vi "OnResize2.vi"(0 "XRef":T15, 1 "Bounds":T13, 2 "Mouse Mods":T11, 3 "State In":T1) -> (14 "Reply":T9, 15 "Fatal Error Out":T8, 16 "State Out":T1)   [LabVIEW 2020, in "Parallel Diagram Block.xnode"]
uses:
  Parallel Diagram Block.xnode
  <vilib>/XNodeSupport/XNodeInt.ctl
  <vilib>/XNodeSupport/NI_XNodeSupport.lvlib
  <vilib>/XNodeSupport/XNodeString.ctl
  <vilib>/XNodeSupport/XNodeStringArray.ctl
  <vilib>/XNodeSupport/XNodeXNodeRef.ctl
  <vilib>/XNodeSupport/XNodeRect32.ctl
  <vilib>/XNodeSupport/XNodeBool.ctl
  <vilib>/XNodeSupport/XNodeMouseMods.ctl
  <vilib>/XNodeSupport/XNodeErrorCluster.ctl
  State.ctl
  Parallel Block/Value Type.ctl
  Parallel Block/Parallel Block.lvlib
  Parallel Block/Type Descriptor.ctl
  <vilib>/picture/picture.llb/imagedata.ctl
  Parallel Block/Direction.ctl
  Parallel Block/Terminal Mode.ctl
  Parallel Block/Terminal Type.ctl
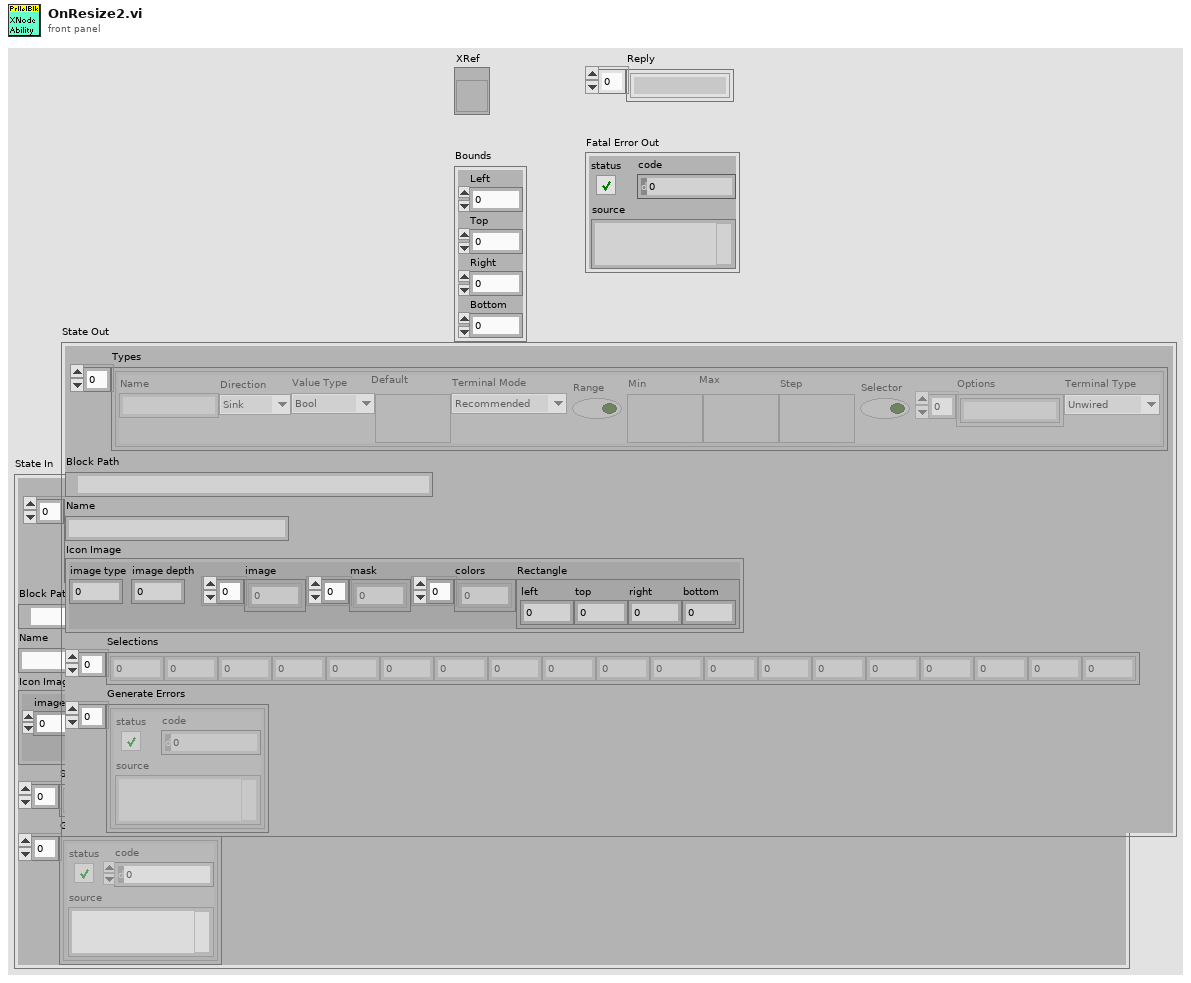
[diagram p1: front panel]
types:
  T1 = typedef "Parallel Diagram Block.xnode/State.ctl" = cluster{"Types":T2[], "Block Path":path, "Name":string, "Icon Image":T7, "Selections":i32[], "Generate Errors":errorcluster[]}
  T2 = typedef "Parallel Block.lvlib/Type Descriptor.ctl" = cluster{"Name":string, "Direction":T3, "Value Type":T4, "Default":variant, "Terminal Mode":T5, "Range":bool, "Min":variant, "Max":variant, "Step":variant, "Selector":bool, "Options":string[], "Terminal Type":T6}
  T3 = typedef "Parallel Block.lvlib/Direction.ctl" = enum16{"Sink", "Source"}
  T4 = typedef "Parallel Block.lvlib/Value Type.ctl" = enum16{"Unknown", "Bool", "U8", "U16", "U32", "U64", "I8", "I16", "I32", "I64", "SGL", "DBL", "CSG", "CDB", "CDBWfm", "String", "DBLWfm"}
  T5 = typedef "Parallel Block.lvlib/Terminal Mode.ctl" = enum16{"Recommended", "Required", "None"}
  T6 = typedef "Parallel Block.lvlib/Terminal Type.ctl" = enum16{"Unwired", "BadType", "Connection", "Value", "Control Ref", "BadRefType"}
  T7 = typedef "imagedata.ctl" = cluster{"image type":i32, "image depth":i32, "image":u8[], "mask":u8[], "colors":u32[], "Rectangle":cluster{"left":i16, "top":i16, "right":i16, "bottom":i16}}
  T8 = typedef "NI_XNodeSupport.lvlib/XNodeErrorCluster.ctl" = errorcluster
  T9 = typedef "NI_XNodeSupport.lvlib/XNodeStringArray.ctl" = T10[]
  T10 = typedef "NI_XNodeSupport.lvlib/XNodeString.ctl" = string
  T11 = typedef "NI_XNodeSupport.lvlib/XNodeMouseMods.ctl" = cluster{"Shift?":T12, "Menu?":T12, "Alt?":T12}
  T12 = typedef "NI_XNodeSupport.lvlib/XNodeBool.ctl" = bool
  T13 = typedef "NI_XNodeSupport.lvlib/XNodeRect32.ctl" = cluster{"Left":T14, "Top":T14, "Right":T14, "Bottom":T14}
  T14 = typedef "NI_XNodeSupport.lvlib/XNodeInt.ctl" = i32
  T15 = typedef "NI_XNodeSupport.lvlib/XNodeXNodeRef.ctl" = refnum<vi>
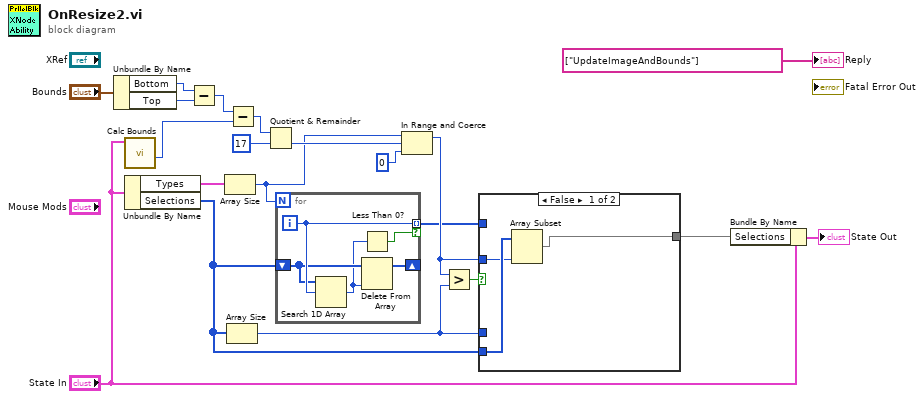
[diagram p0: block diagram]
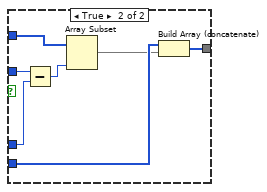
[diagram p2: hidden frame]
diagram:
  n1 = Unbundle By Name("Bounds") -> ("Bottom"=w19:T14, "Top"=w18:T14)
  n2 = call "Calc Bounds.vi"("State"="State In") -> ("Collapsed"=w8:i32)  [unwired: 6 in, 4 out]
  n3 = Unbundle By Name("State In") -> ("Types"=w12:T2[], "Selections"=w2:i32[])
  n4 = Subtract(x=w19, y=w18) -> (x-y=w17:T14)
  n5 = Array Size(array=w12) -> (size(s)=w3:i32)
  n6 = Array Size(array=w2) -> (size(s)=w6:i32)
  n7 = Subtract(x=w17, y=w8) -> (x-y=w16:T14)
  n8 = Quotient & Remainder(x=w16, y=T14 17) -> (floor(x/y)=w10:T14)  [unwired: 1 out]
  n9 = for {
    N: w3 -> [_]
    tunnel: [w25] -> w1 mode=indexing if=w21
    shift-right: [w23] -> _
    shift-left: w2 -> [w24]
    i -> [w25]
    n10 = Search 1D Array(1D array=w24, element=w25) -> (index of element=w22:i32)  [unwired: 1 in]
    n11 = Less Than 0?(x=w22) -> (x < 0?=w21:bool)
    n12 = Delete From Array(array=w24, index=w22) -> (array with subset deleted=w23:i32[])  [unwired: 1 in, 1 out]
  }
  n13 = In Range and Coerce(upper limit=w3, x=w10, lower limit=0 ("Expanded Count")) -> (coerced(x)=w5:T14)  [unwired: 1 out]
  n14 = Greater?(x=w5, y=w6) -> (0:w7:bool)
  n15 = case shown="False" w7 {
    tunnel: w6 -> [_ w34]
    tunnel: w5 -> [w27 w35]
    tunnel: w2 -> [w28 w33]
    tunnel: [w26 w32] -> w4
    tunnel: w1 -> [_ w31]
    frame False {
      n16 = Array Subset(array=w28, length=w27) -> (w26:i32[])  [unwired: 1 in]
    }
    frame True {
      n17 = Subtract(x=w35, y=w34) -> (x-y=w30:T14)
      n18 = Array Subset(array=w31, length=w30) -> (w29:i32[])  [unwired: 1 in]
      n19 = Build Array (concatenate)(w33, w29) -> (w32:i32[])
    }
  }
  n20 = Bundle By Name(cluster="State In", "Selections"=w4) -> (→"State Out":T1)
  "Reply" <- T9 ["UpdateImageAndBounds"] ("Reply")
